vi "Initialise_Single_Puff.vi"() -> (5 "Plug in titles":string[](array[string]), 7 "Plug in values":string[](array[string]))   [LabVIEW 2012]
uses:
  Controls/Post_Process.ctl
  Controls/Setup.ctl
  Globals/Meas_global.vi
panel:
  in  "Initial Purge (s)":u32=7
  out "Case Currently On":string="Set Acquisition interlock"
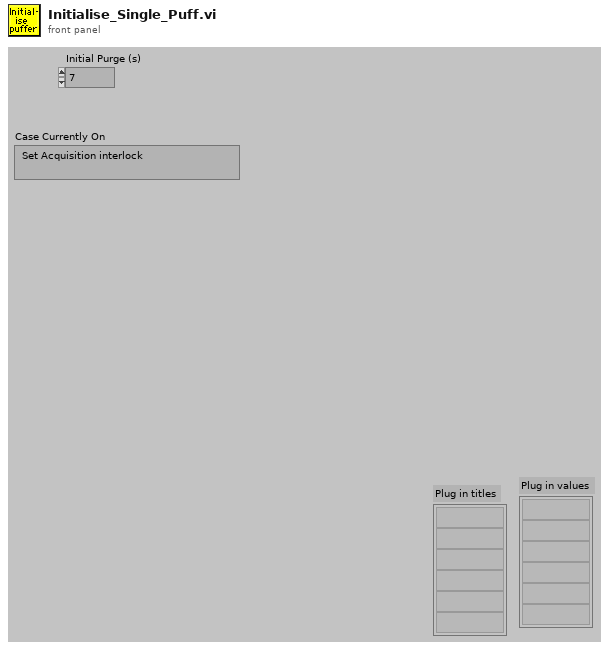
[diagram p1: front panel]
types:
  T1 = typedef "Setup.ctl" = enum16{"Run Program", "Show Setup", "Save Current Setup", "Setup Front Panel"}
  T2 = typedef "Post_Process.ctl" = enum16{"Take New Data", "Post Process Raw Data File"}
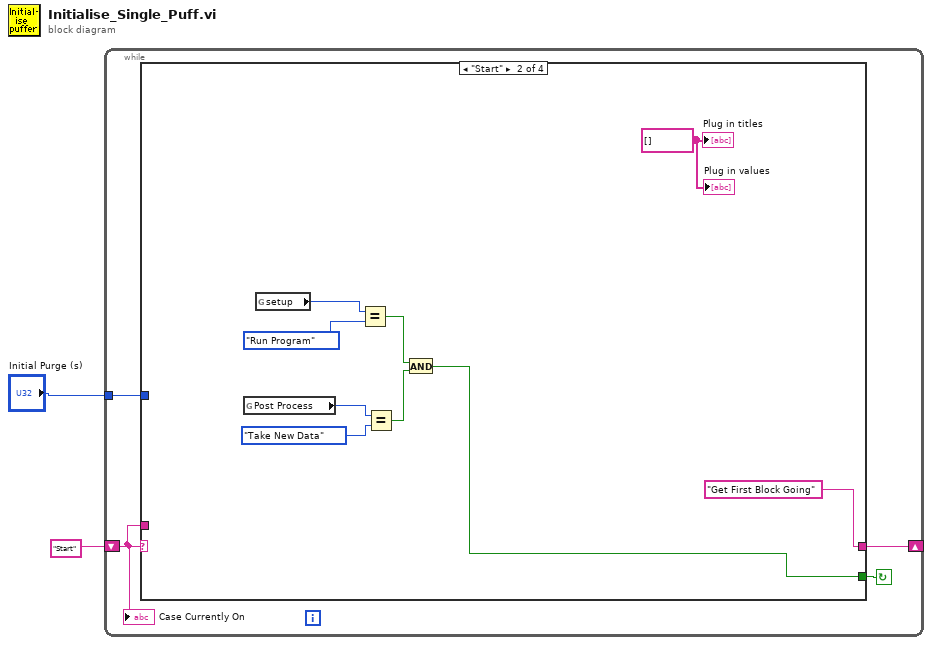
[diagram p0: block diagram]
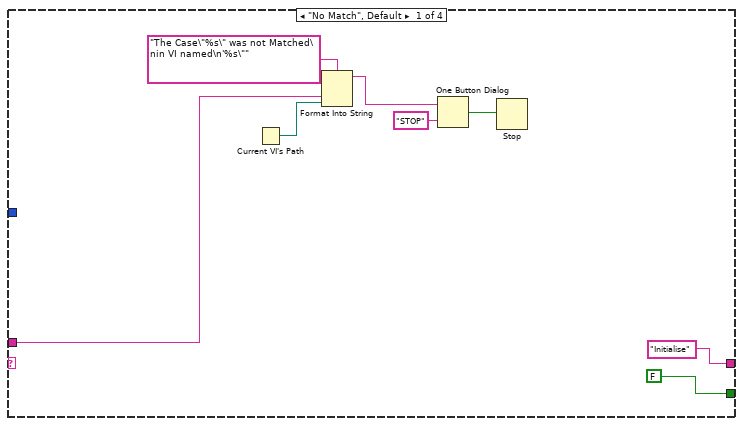
[diagram p2: hidden frame]
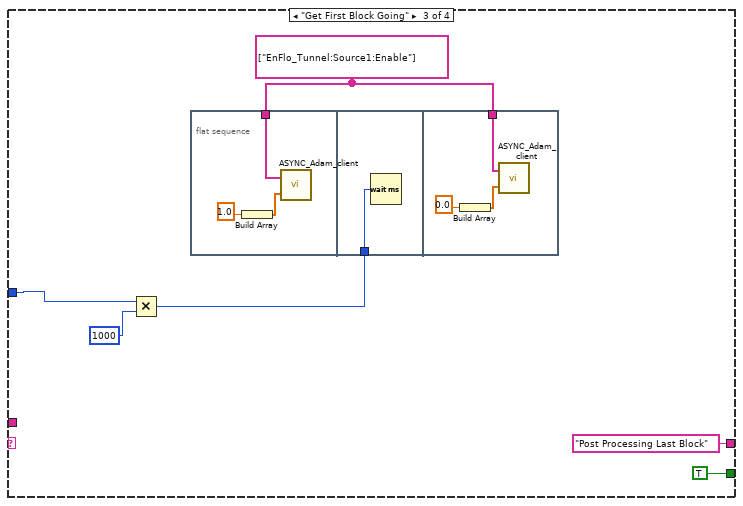
[diagram p3: hidden frame]
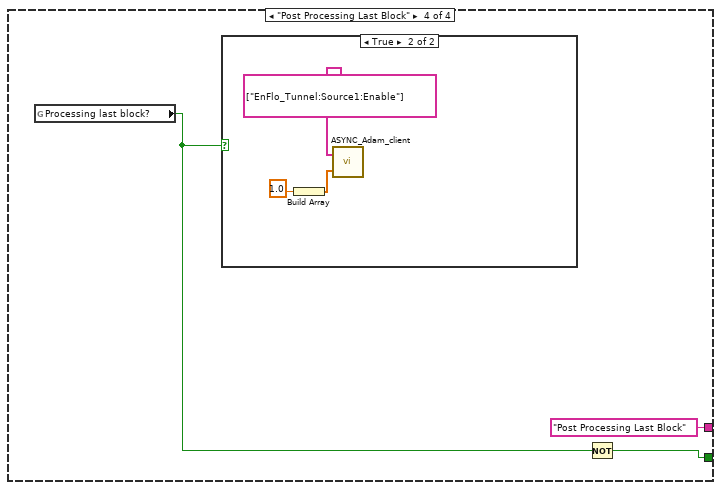
[diagram p4: hidden frame]
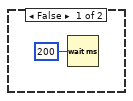
[diagram p5: hidden frame]
diagram:
  n1 = while {
    shift-left: "Start" -> [w4]
    shift-right: [w5] -> _
    tunnel: "Initial Purge (s)" -> [w3]
    stop <- w6 continue-if-true
    n2 = case shown="\"Start\"" w4 {
      tunnel: [FALSE w15 TRUE ("Command Found") w37] -> w6
      tunnel: ["Initialise" "Get First Block Going" "Post Processing Last Block" "Post Processing Last Block"] -> w5
      tunnel: w4 -> [w9 _ _ _]
      tunnel: w3 -> [_ _ w27 _]
      frame "No Match", Default {
        n3 = Current VI's Path() -> (path=w8:path)
        n4 = Format Into String(format string="The Case\"%s\" was not Matched\nin VI named\n'%s\"" ("Format String"), w9, w8) -> (resulting string=w12:string)  [unwired: 2 in, 1 out]
        n5 = One Button Dialog(message=w12, button name ("OK")="STOP") -> (true=w10:bool)
        n6 = Stop(stop? (T)=w10) -> ()
      }
      frame "Start" {
        w21 = string[] [] ("Plug in titles")
        n7 = global read "Meas_global.vi" "Post Process"() -> (w20:T2)
        n8 = global read "Meas_global.vi" "setup"() -> (w22:T1)
        n9 = Equal?(x=w22, y=Setup."Run Program") -> (x = y?=w16:bool)
        n10 = Equal?(x=w20, y=Post_Process."Take New Data" ("Post Process")) -> (x = y?=w17:bool)
        n11 = And(x=w16, y=w17) -> (x .and. y?=w15:bool)
        "Plug in values" <- w21
        "Plug in titles" <- w21
      }
      frame "Get First Block Going" {
        w24 = string[] ["EnFlo_Tunnel:Source1:Enable"] ("appended array")
        n12 = Multiply(x=w27, y=u32 1000) -> (x*y=w25:u32)
        n13 = flat-sequence {
          tunnel: w24 -> [w30]
          tunnel: w25 -> [w33]
          tunnel: w24 -> [w34]
          frame #0 {
            n14 = Build Array(1.0 ("New Value")) -> (w32:dbl[])
            n15 = call "ASYNC_Adam_client.vi"("Values"=w32, "Channel Names"=w30) -> ()  [unwired: 2 out]
          }
          frame #1 {
            n16 = Wait (ms)(milliseconds to wait=w33) -> ()  [unwired: 1 out]
          }
          frame #2 {
            n17 = Build Array(0.0 ("New Value")) -> (w35:dbl[])
            n18 = call "ASYNC_Adam_client.vi"("Values"=w35, "Channel Names"=w34) -> ()  [unwired: 2 out]
          }
        }
      }
      frame "Post Processing Last Block" {
        n19 = global read "Meas_global.vi" "Processing last block?"() -> (w38:bool)
        n20 = case shown="True" w38 {
          frame False {
            n21 = Wait (ms)(milliseconds to wait=u32 200) -> ()  [unwired: 1 out]
          }
          frame True {
            n22 = Build Array(1.0 ("New Value")) -> (w41:dbl[])
            n23 = call "ASYNC_Adam_client.vi"("Values"=w41, "Channel Names"=string[] ["EnFlo_Tunnel:Source1:Enable"] ("appended array")) -> ()  [unwired: 2 out]
          }
        }
        n24 = Not(x=w38) -> (.not. x?=w37:bool)
      }
    }
    "Case Currently On" <- w4
  }
